vi "calc-velocities.vi"(8 "Y in":dbl[](array[numeric])=[1.0, -0.4999999999999998, -0.5000000000000004, 1.0], 9 "Radius":dbl=2000.0, 10 "Velocidade (mm/s)":ext=0.05, 11 "X in":dbl[](array[numeric])=[0.0, 0.8660254037844387, -0.8660254037844384, 0.0]) -> (0 "Vy":ext[](array[numeric])=[0.04330127018922192983, 1.9691137908567695728e-17, 0.04330127018922193538], 1 "Vx":ext[](array[numeric])=[0.025000000000000005552, 0.05, 0.024999999999999986123], 2 "Y":dbl[](array[numeric])=[2000.0, -999.9999999999995, -1000.0000000000009, 2000.0], 3 "X":dbl[](array[numeric])=[0.0, 1732.0508075688774, -1732.0508075688767, 0.0], 4 "Delta Y":dbl[](array[numeric])=[-2999.9999999999995, -1.3642420526593924e-12, 3000.000000000001], 5 "Delta X":dbl[](array[numeric])=[1732.0508075688774, -3464.1016151377544, 1732.0508075688767])   [LabVIEW 2014]
doc: "André Romero - 2018\nandretec@ifsc.usp.br"
panel:
  out "array w/ subset deleted 2":dbl[](array[numeric])=[-999.9999999999995, -1000.0000000000009, 2000.0]
  out "array w/ subset deleted":ext[](array[numeric])=[1732.0508075688774, -1732.0508075688767, 0.0]
  out "XY Graph 2":cluster{dbl[], dbl[]}(graph)={[0.0, 1732.0508075688774, -1732.0508075688767, 0.0], [2000.0, -999.9999999999995, -1000.0000000000009, 2000.0]}
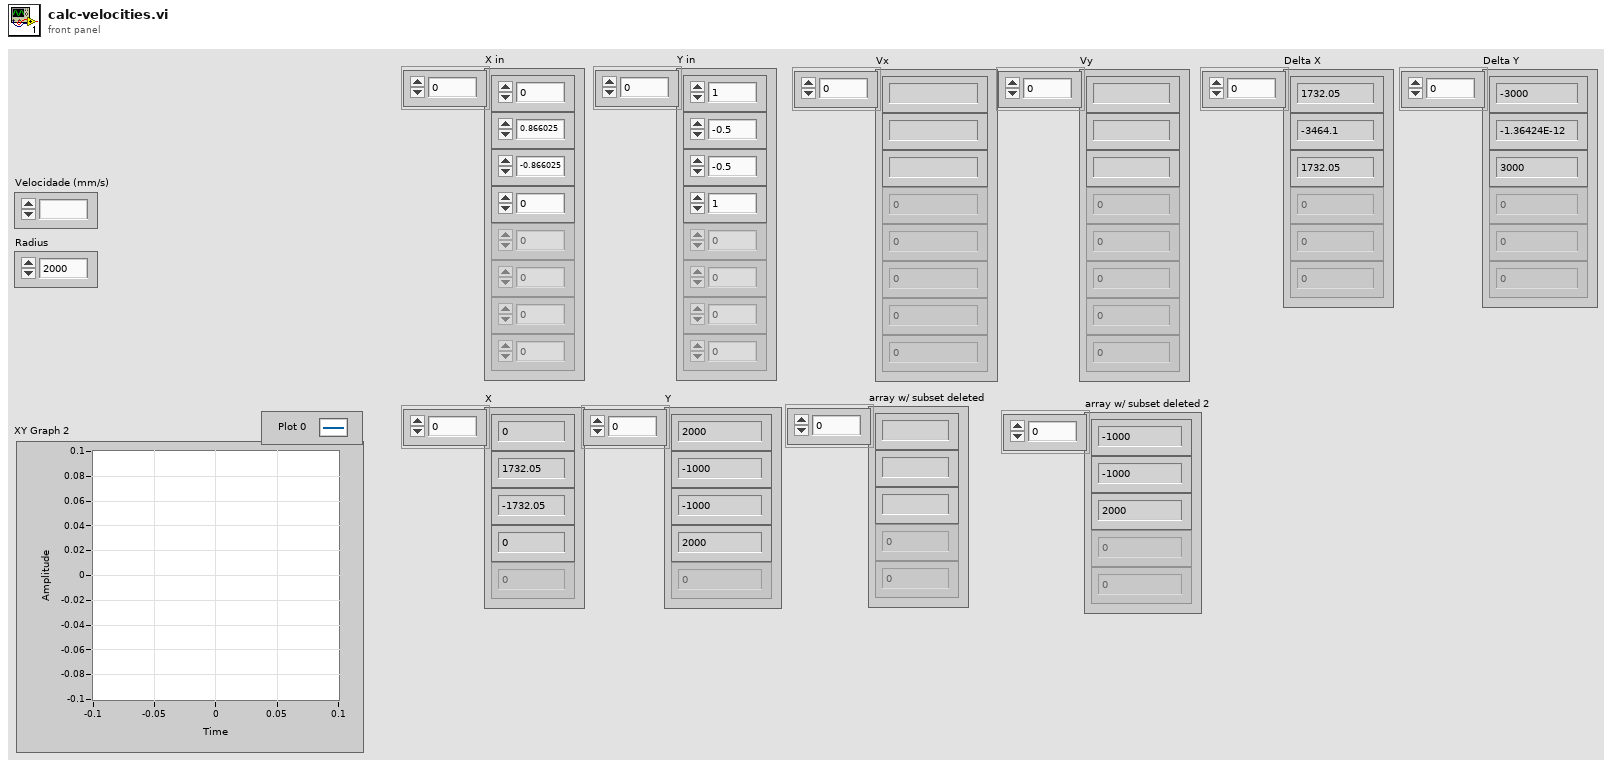
[diagram p1: front panel]
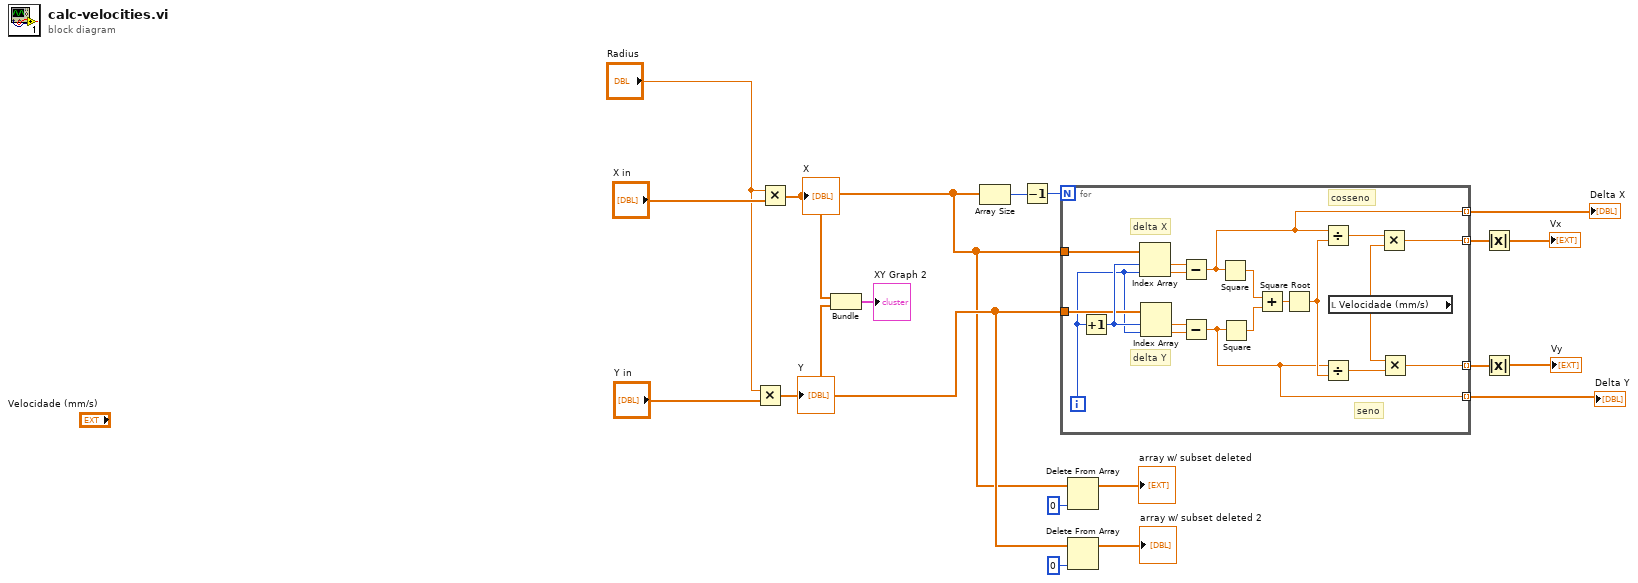
[diagram p0: block diagram]
diagram:
  n1 = Multiply(x="Radius", y="Y in") -> (x*y=w6:dbl[])
  "Y" <- w6
  n2 = Multiply(x="Radius", y="X in") -> (x*y=w5:dbl[])
  "X" <- w5
  n3 = Bundle(w5, w6) -> (→"XY Graph 2":cluster{dbl[], dbl[]})  [unwired: 1 in]
  n4 = Array Size(array=w5) -> (size(s)=w14:i32)
  n5 = Decrement(x=w14) -> (x-1=w11:i32)
  n6 = for {
    N: w11 -> [_]
    tunnel: w5 -> [w26]
    tunnel: w6 -> [w25]
    tunnel: [w23] -> w13 mode=indexing
    tunnel: [w22] -> w12 mode=indexing
    tunnel: [w21] -> w4 mode=indexing
    tunnel: [w20] -> w3 mode=indexing
    i -> [w24]
    # "seno"
    # "cosseno"
    # "delta Y"
    # "delta X"
    n7 = Increment(x=w24) -> (x+1=w37:i32)
    n8 = Index Array(array=w26, index #1=w37, index #2=w24) -> (element #1=w28:dbl, element #2=w35:dbl)
    n9 = Index Array(array=w25, index #1=w37, index #2=w24) -> (element #1=w27:dbl, element #2=w36:dbl)
    n10 = Subtract(x=w28, y=w35) -> (x-y=w21:dbl)
    n11 = Subtract(x=w27, y=w36) -> (x-y=w20:dbl)
    n12 = Square(x=w21) -> (x^2=w34:dbl)
    n13 = Square(x=w20) -> (x^2=w33:dbl)
    n14 = Add(x=w34, y=w33) -> (x+y=w32:dbl)
    n15 = Square Root(x=w32) -> (sqrt(x)=w31:dbl)
    n16 = Divide(x=w21, y=w31) -> (x/y=w30:dbl)
    n17 = Divide(x=w20, y=w31) -> (x/y=w29:dbl)
    n18 = local read "Velocidade (mm/s)"() -> (w19:ext)
    n19 = Multiply(x=w30, y=w19) -> (x*y=w23:ext)
    n20 = Multiply(x=w19, y=w29) -> (x*y=w22:ext)
  }
  "Delta X" <- w4
  "Delta Y" <- w3
  n21 = Delete From Array(array=w5, index=0) -> (array with subset deleted=→"array w/ subset deleted":dbl[])  [unwired: 1 in, 1 out]
  n22 = Delete From Array(array=w6, index=0) -> (array with subset deleted=→"array w/ subset deleted 2":dbl[])  [unwired: 1 in, 1 out]
  n23 = Absolute Value(x=w13) -> (abs(x)=→"Vx":ext[])
  n24 = Absolute Value(x=w12) -> (abs(x)=→"Vy":ext[])
